vi "A5114-2.vi"(10 "device_id":u8=23 min=1 max=99 format="%02d", 11 "Comport":refnum<visa-resource-name>="COM3") -> (1 "Volt_data":string, 2 "check_Sum_OK":bool, 3 "Is_Estb_Communication_OK":bool)   [LabVIEW 2011]
panel:
  out "dev_ID_L":u8 format="%x"
  out "dev_ID_H":u8 format="%x"
  out "ID byte array":u8[](array[numeric]) format="%x"
  out "bytes read":u32
  in  "Release Link CMD":u8[](array[numeric])=[4, 13, 10] format="%x"
  out "BCC_H":u8 format="%x"
  out "BCC_L":u8 format="%x"
  out "Byte_BCC":u32 format="%x"
  out "number_loop":i32
  out "length_ret_mes":i32
  out "ret_mes_byte":u8[](array[numeric]) format="%x"
  out "ret_mes":string
  in  "CMD_MES":u8[](array[numeric])=[2, 77, 69, 83, 3, 56, 69, 13, 10] format="%x"
  out "LF":u8 format="%x"
  out "CR":u8 format="%x"
  out "ID_L":u8 format="%x"
  out "ID_H":u8 format="%x"
  out "ACK":u8 format="%x"
  out "read string":string
  out "string_WR":string
  in  "Establishing Communication CMD":u8[](array[numeric])=[5, 50, 51, 13, 10] format="%x"
  out "Resp_Estab_cmd":u8[](array[numeric]) format="%x"
  # "Send Command For Establishing Communication link"
  # "Send Command to Panel Meter for Measurement Volt"
  # "STX"
  # "STX"
  # "ENQ"
  # "M"
  # "E"
  # "S"
  # "CR"
  # "ETX"
  # "LF"
  # "BCC_H"
  # "BCC_L"
  # "CR"
  # "LF"
  # "ETX"
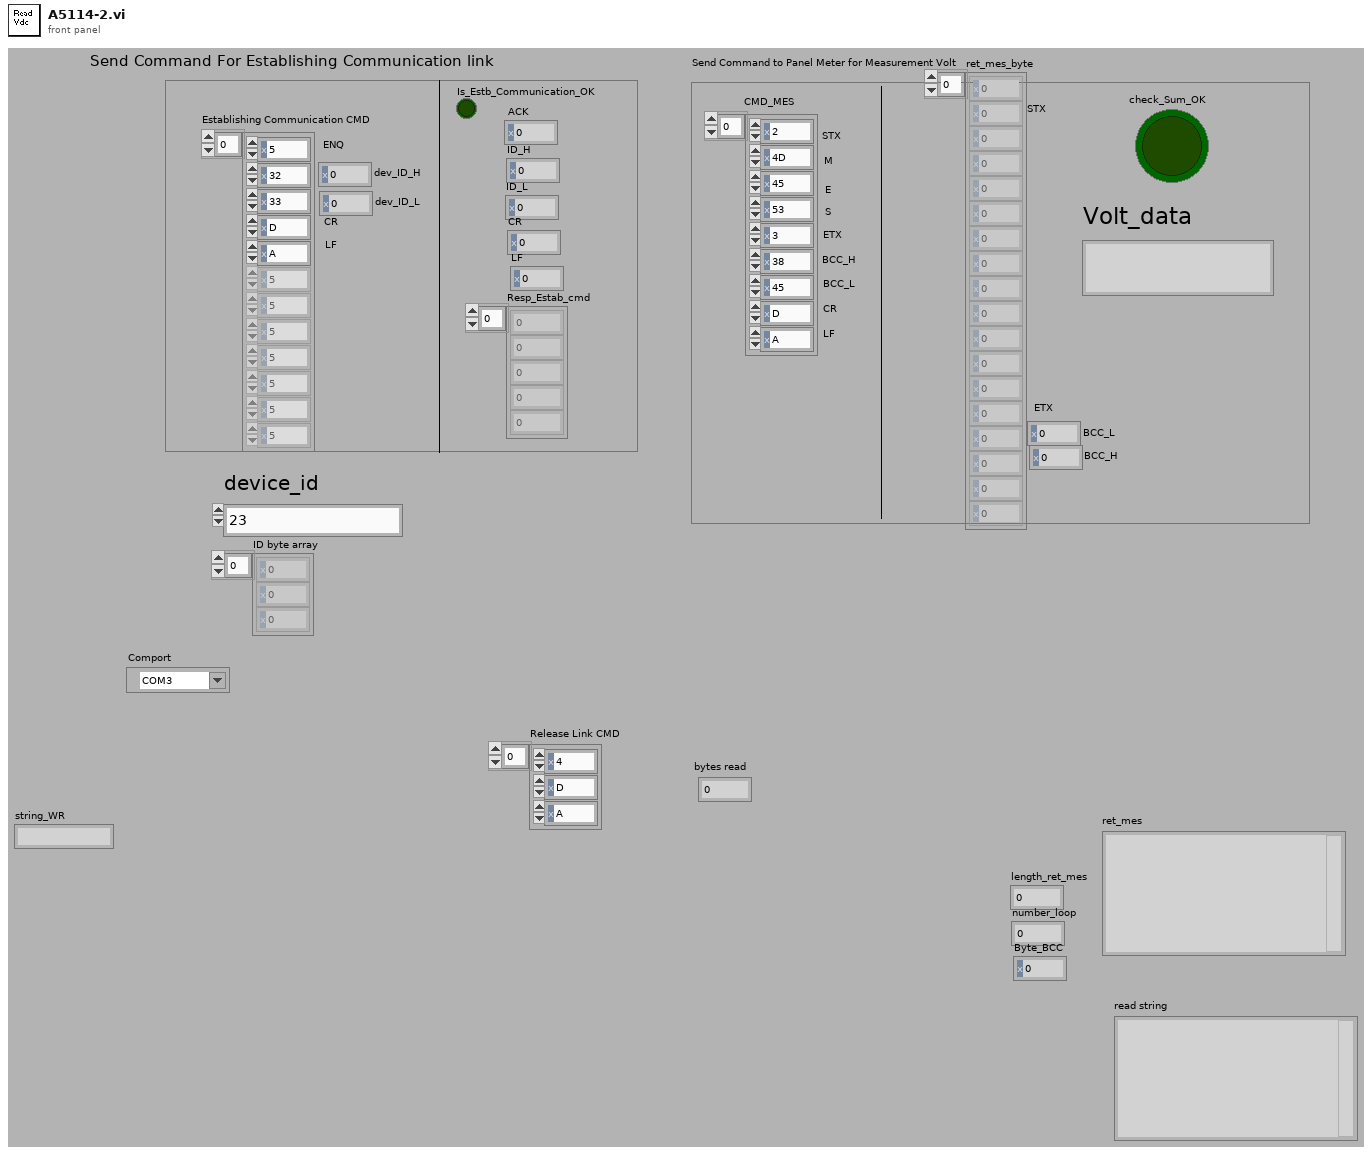
[diagram p1: front panel]
types:
  T1 = enum8{"Measurement", "Calculate_checksum", "detect_checksum", "END"}
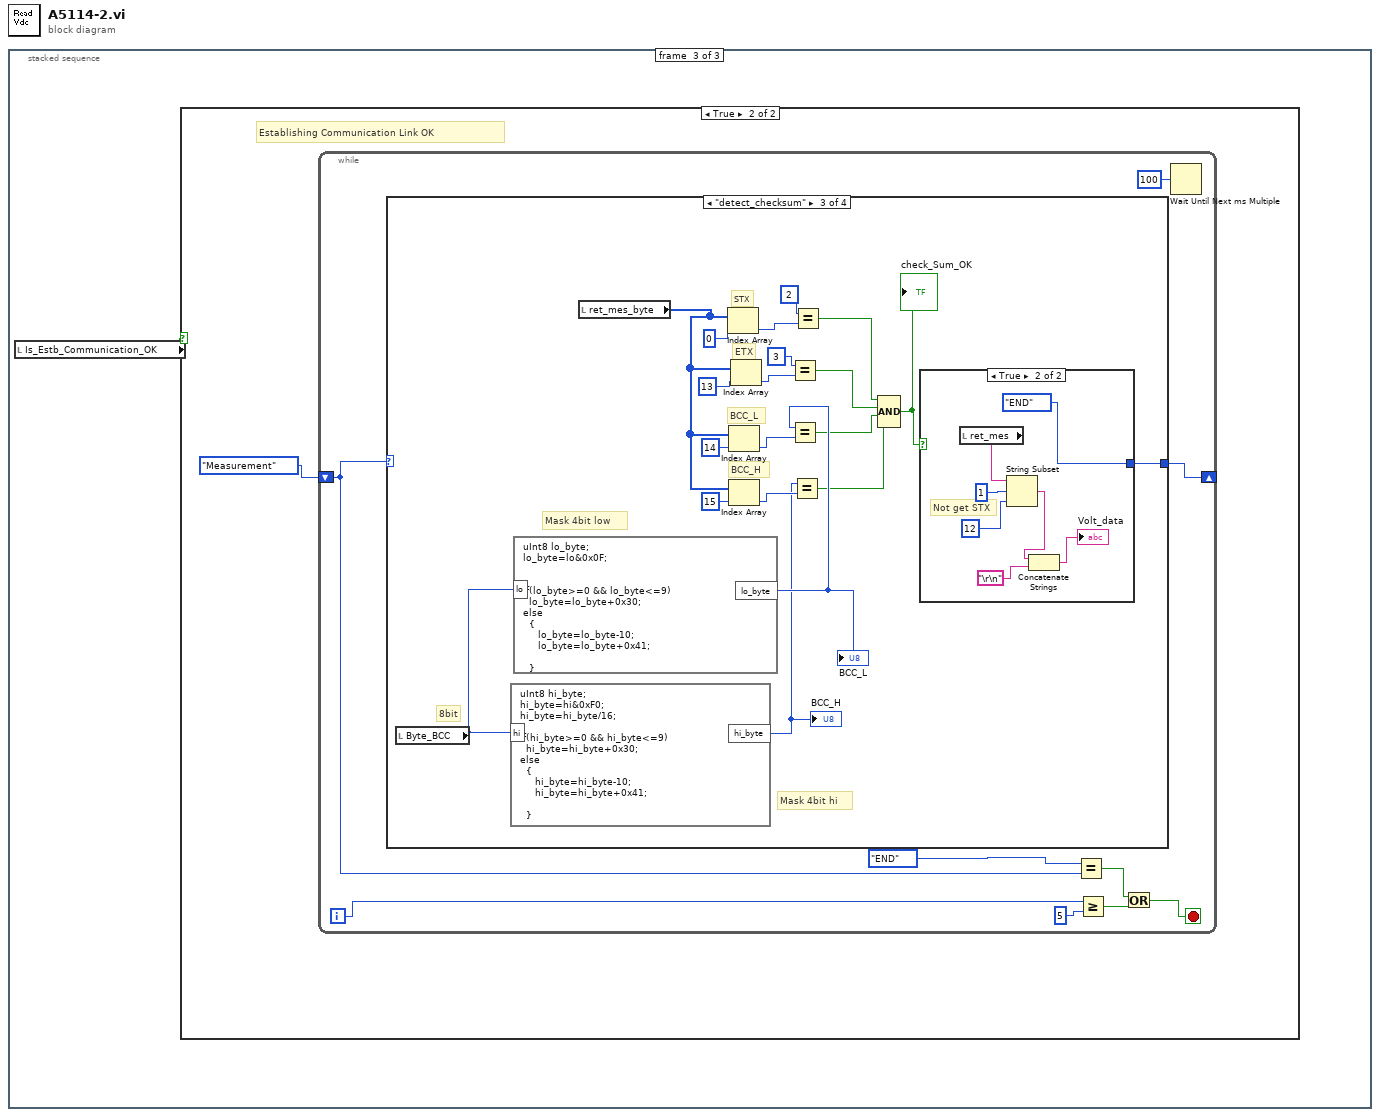
[diagram p0: block diagram]
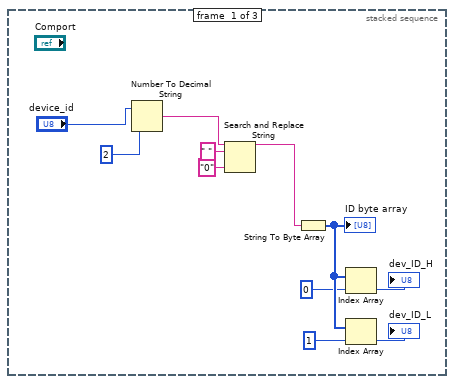
[diagram p2: hidden frame]
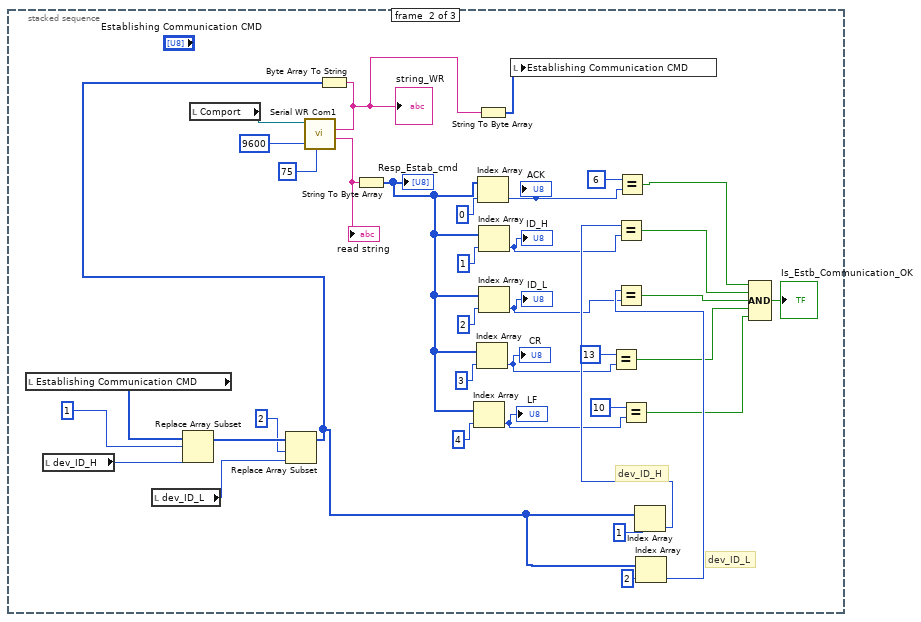
[diagram p3: hidden frame]
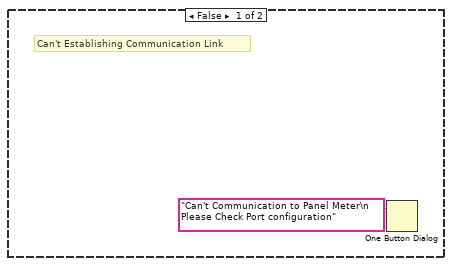
[diagram p4: hidden frame]
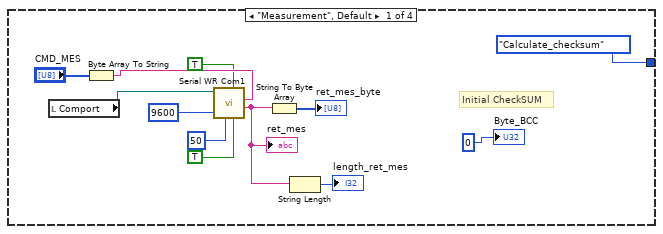
[diagram p5: hidden frame]
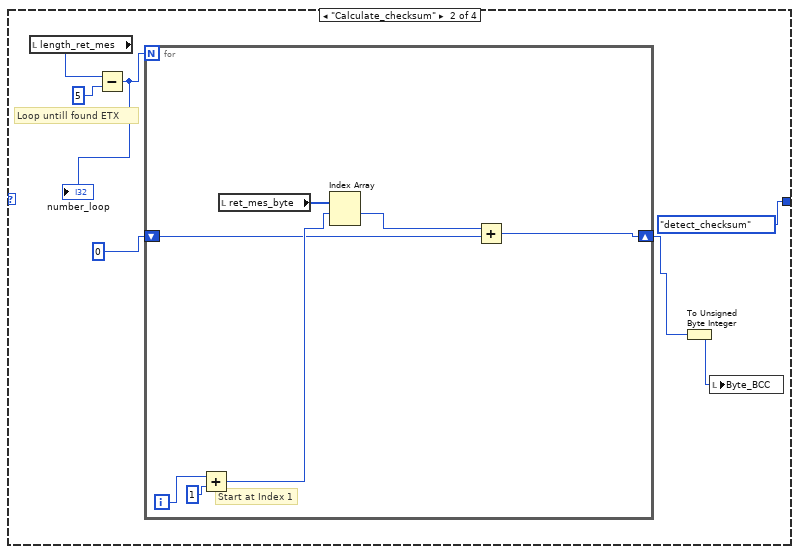
[diagram p6: hidden frame]
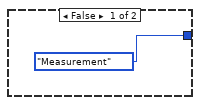
[diagram p7: hidden frame]
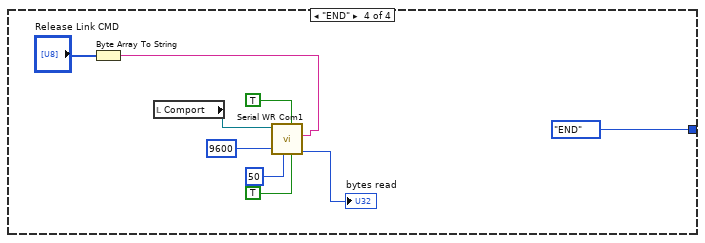
[diagram p8: hidden frame]
diagram:
  n1 = stacked-sequence {
    frame #0 {
      n2 = Number To Decimal String(number="device_id", width (-)=i16 2) -> (decimal integer string=w9:string)
      n3 = Search and Replace String(input string=w9, search string=" ", replace string="0" ("replace string (\"\")")) -> (result string=w6:string)  [unwired: 1 in, 7 out]
      n4 = String To Byte Array(string=w6) -> (unsigned byte array=w5:u8[])
      "ID byte array" <- w5
      n5 = Index Array(array=w5, index=0) -> (element=→"dev_ID_H":u8)
      n6 = Index Array(array=w5, index=1) -> (element=→"dev_ID_L":u8)
    }
    frame #1 {
      # "dev_ID_L"
      # "dev_ID_H"
      n7 = local read "Establishing Communication CMD"() -> (w21:u8[])
      n8 = local read "dev_ID_H"() -> (w19:u8)
      n9 = local read "dev_ID_L"() -> (w17:u8)
      n10 = Replace Array Subset(array=w21, new element=w19, index=1) -> (w18:u8[])
      n11 = local read "Comport"() -> (w12:refnum<visa-resource-name>)
      n12 = Replace Array Subset(array=w18, new element=w17, index=2) -> (w13:u8[])
      n13 = Byte Array To String(unsigned byte array=w13) -> (string=w14:string)
      "string_WR" <- w14
      n14 = call "Serial WR Com1.vi"("string to write"=w14, "delay before read (ms)"=u32 75, "baud rate"=u32 9600, "VISA resource name"=w12) -> ("read string"=w48:string)  [unwired: 6 in, 1 out]
      "read string" <- w48
      n15 = String To Byte Array(string=w48) -> (unsigned byte array=w40:u8[])
      "Resp_Estab_cmd" <- w40
      n16 = Index Array(array=w40, index=4) -> (element=w28:u8)
      "LF" <- w28
      n17 = Index Array(array=w40, index=3) -> (element=w30:u8)
      "CR" <- w30
      n18 = String To Byte Array(string=w14) -> (unsigned byte array=w15:u8[])
      n19 = Index Array(array=w40, index=0) -> (element=w39:u8)
      "ACK" <- w39
      n20 = Index Array(array=w40, index=1) -> (element=w34:u8)
      "ID_H" <- w34
      n21 = Index Array(array=w40, index=2) -> (element=w32:u8)
      "ID_L" <- w32
      n22 = local write "Establishing Communication CMD"(w15) -> ()
      n23 = Equal?(x=u8 13, y=w30) -> (x = y?=w23:bool)
      n24 = Equal?(x=u8 6, y=w39) -> (x = y?=w27:bool)
      n25 = Equal?(x=u8 10, y=w28) -> (x = y?=w24:bool)
      n26 = Index Array(array=w13, index=1) -> (element=w35:u8)
      n27 = Equal?(x=w35, y=w34) -> (x = y?=w26:bool)
      n28 = Index Array(array=w13, index=2) -> (element=w33:u8)
      n29 = Equal?(x=w33, y=w32) -> (x = y?=w25:bool)
      n30 = Compound Arithmetic op=AND(w27, w26, w25, w23, w24) -> (→"Is_Estb_Communication_OK":bool)
    }
    frame #2 {
      n31 = local read "Is_Estb_Communication_OK"() -> (w49:bool)
      n32 = case shown="True" w49 {
        frame False {
          # "Can't Establishing Communication Link"
          n33 = One Button Dialog(message="Can't Communication to Panel Meter\n Please Check Port configuration") -> ()  [unwired: 2 out]
        }
        frame True {
          # "Establishing Communication Link OK"
          n34 = while {
            shift-right: [w53] -> _
            shift-left: T1."Measurement" -> [w54]
            i -> [w56]
            stop <- w58 stop-if-true
            n35 = case shown="\"detect_checksum\"" w54 {
              tunnel: [T1."Calculate_checksum" T1."detect_checksum" w93 T1."END"] -> w53
              frame "Measurement", Default {
                # "Initial CheckSUM"
                n36 = local read "Comport"() -> (w61:refnum<visa-resource-name>)
                n37 = Byte Array To String(unsigned byte array="CMD_MES") -> (string=w69:string)
                n38 = call "Serial WR Com1.vi"("string to write"=w69, "read"=TRUE, "write"=TRUE, "delay before read (ms)"=u32 50, "baud rate"=u32 9600, "VISA resource name"=w61) -> ("read string"=w66:string)  [unwired: 4 in, 1 out]
                "ret_mes" <- w66
                n39 = String To Byte Array(string=w66) -> (unsigned byte array=→"ret_mes_byte":u8[])
                n40 = String Length(string=w66) -> (length=→"length_ret_mes":i32)
                "Byte_BCC" <- u32 0 ("Byte_BCC")
              }
              frame "Calculate_checksum" {
                # "Loop untill found ETX"
                n41 = local read "length_ret_mes"() -> (w78:i32)
                n42 = Subtract(x=w78, y=5) -> (x-y=w79:i32)
                "number_loop" <- w79
                n43 = for {
                  N: w79 -> [_]
                  shift-right: [w82] -> w74
                  shift-left: 0 -> [w81]
                  i -> [w85]
                  # "Start at Index 1"
                  n44 = Add(x=w85, y=1) -> (x+y=w83:i32)
                  n45 = local read "ret_mes_byte"() -> (w86:u8[])
                  n46 = Index Array(array=w86, index #1=w83) -> (element #1=w80:u8)  [unwired: 1 in, 1 out]
                  n47 = Add(x=w80, y=w81) -> (x+y=w82:i32)
                }
                n48 = To Unsigned Byte Integer(number=w74) -> (unsigned 8bit integer=w73:u8)
                n49 = local write "Byte_BCC"(w73) -> ()
              }
              frame "detect_checksum" {
                # "Mask 4bit hi"
                # "Mask 4bit low"
                # "8bit"
                # "ETX"
                # "BCC_H"
                # "BCC_L"
                # "STX"
                n50 = local read "Byte_BCC"() -> (w87:u32)
                n51 = formula code="uInt8 hi_byte;\nhi_byte=hi&0xF0;\nhi_byte=hi_byte/16;\n\nif(hi_byte>=0 && hi_byte<=9)\n  hi_byte=hi_byte+0x30;\nelse\n  {\n     hi_byte=hi_byte-10; \n     hi_byte=hi_byte+0x41; \n\n  }"("hi"=w87) -> ("hi_byte"=w88:u8)
                "BCC_H" <- w88
                n52 = formula code="uInt8 lo_byte;\nlo_byte=lo&0x0F;\n\n\nif(lo_byte>=0 && lo_byte<=9)\n  lo_byte=lo_byte+0x30;\nelse\n  {\n     lo_byte=lo_byte-10; \n     lo_byte=lo_byte+0x41; \n\n  }"("lo"=w87) -> ("lo_byte"=w99:u8)
                "BCC_L" <- w99
                n53 = local read "ret_mes_byte"() -> (w106:u8[])
                n54 = Index Array(array=w106, index=0) -> (element=w105:u8)
                n55 = Index Array(array=w106, index=14) -> (element=w103:u8)
                n56 = Index Array(array=w106, index=15) -> (element=w102:u8)
                n57 = Index Array(array=w106, index=13) -> (element=w104:u8)
                n58 = Equal?(x=u8 3, y=w104) -> (x = y?=w97:bool)
                n59 = Equal?(x=w99, y=w103) -> (x = y?=w96:bool)
                n60 = Equal?(x=w88, y=w102) -> (x = y?=w95:bool)
                n61 = Equal?(x=u8 2, y=w105) -> (x = y?=w98:bool)
                n62 = Compound Arithmetic op=AND(w98, w97, w96, w95) -> (w94:bool)
                "check_Sum_OK" <- w94
                n63 = case shown="True" w94 {
                  tunnel: [T1."Measurement" T1."END"] -> w93
                  frame False {
                  }
                  frame True {
                    # "Not get STX"
                    n64 = local read "ret_mes"() -> (w114:string)
                    n65 = String Subset(string=w114, offset (0)=1, length (rest)=12 ("length (rest)")) -> (substring=w109:string)
                    n66 = Concatenate Strings(w109, "\r\n") -> (→"Volt_data":string)
                  }
                }
              }
              frame "END" {
                n67 = Byte Array To String(unsigned byte array="Release Link CMD") -> (string=w117:string)
                n68 = local read "Comport"() -> (w115:refnum<visa-resource-name>)
                n69 = call "Serial WR Com1.vi"("string to write"=w117, "read"=TRUE, "write"=TRUE, "delay before read (ms)"=u32 50, "baud rate"=u32 9600, "VISA resource name"=w115) -> ("bytes read"=→"bytes read":u32)  [unwired: 4 in, 1 out]
              }
            }
            n70 = Equal?(x=T1."END", y=w54) -> (x = y?=w59:bool)
            n71 = Greater Or Equal?(x=w56, y=5 ("x")) -> (x >= y?=w60:bool)
            n72 = Or(x=w59, y=w60) -> (x .or. y?=w58:bool)
            n73 = Wait Until Next ms Multiple(millisecond multiple=u32 100) -> ()  [unwired: 1 out]
          }
        }
      }
    }
  }
